vi "freqCruve.vi"(0 "Start":dbl, 1 "End":dbl, 2 "Path":path, 3 "Step":dbl, 4 "error in (no error)":errorcluster) -> (5 "error out":errorcluster)   [LabVIEW 2010]
panel:
  out "WC Amplitude":dbl(graph)
  out "WC Phase Shift":dbl(graph)
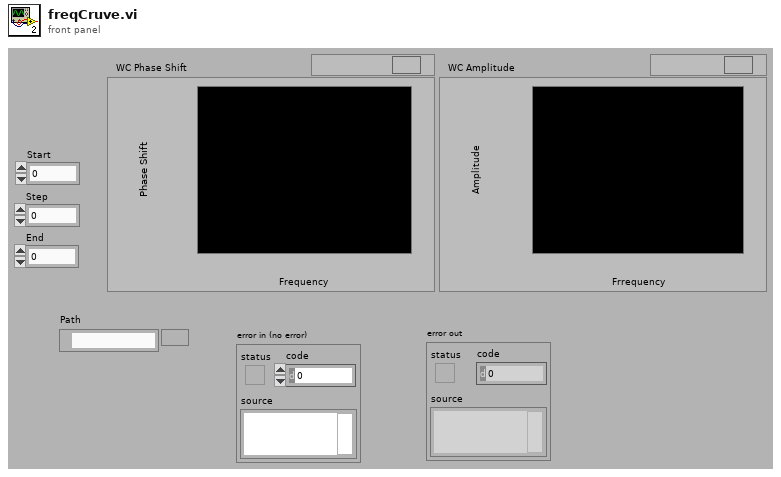
[diagram p1: front panel]
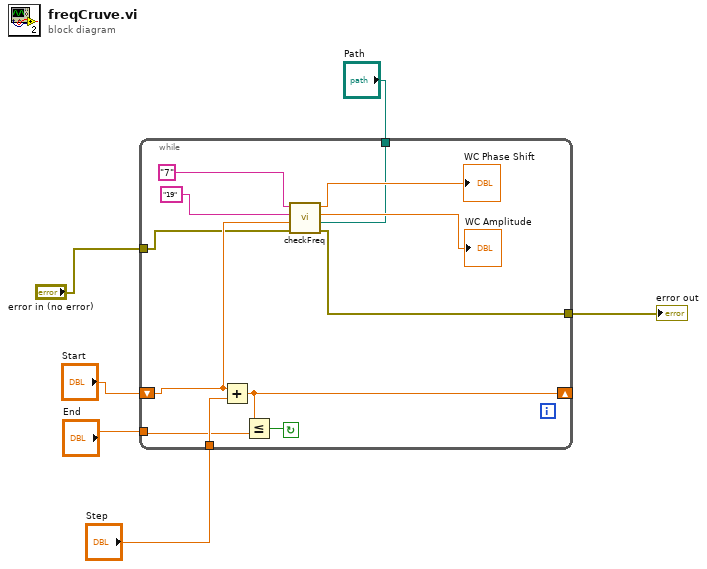
[diagram p0: block diagram]
diagram:
  n1 = while {
    shift-right: [w13] -> _
    shift-left: "Start" -> [w15]
    tunnel: "Step" -> [w18]
    tunnel: "End" -> [w12]
    tunnel: "error in (no error)" -> [w9]
    tunnel: [w8] -> w2
    tunnel: "Path" -> [w7]
    stop <- w14 continue-if-true
    n2 = Add(x=w15, y=w18) -> (x+y=w13:dbl)
    n3 = Less Or Equal?(x=w13, y=w12) -> (x <= y?=w14:bool)
    n4 = call "checkFreq.vi"("Path"=w7, "error in"=w9, "Set Frequency"=w15, "Wave generator"="19", "Lock-In"="7") -> ("error out"=w8:errorcluster, "Amplitude"=→"WC Amplitude":dbl, "Phase Shift"=→"WC Phase Shift":dbl)
  }
  "error out" <- w2
